vi "SeqnRead.vi"(8 "error in (no error)":errorcluster, 11 "File in":path) -> (0 "error out":errorcluster, 1 "Cohort List":cluster{string, i32}[](array[cluster]), 2 "Seqn out":refnum<class "Sequence.lvclass">)   [LabVIEW 2012, in "Sequence.lvclass"]
uses:
  Sequence.lvclass
  Cohort.lvclass
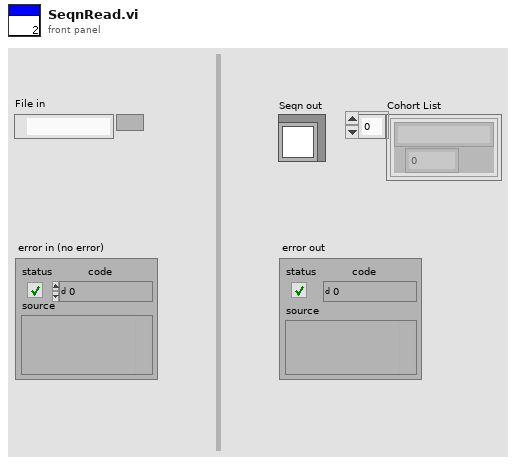
[diagram p1: front panel]
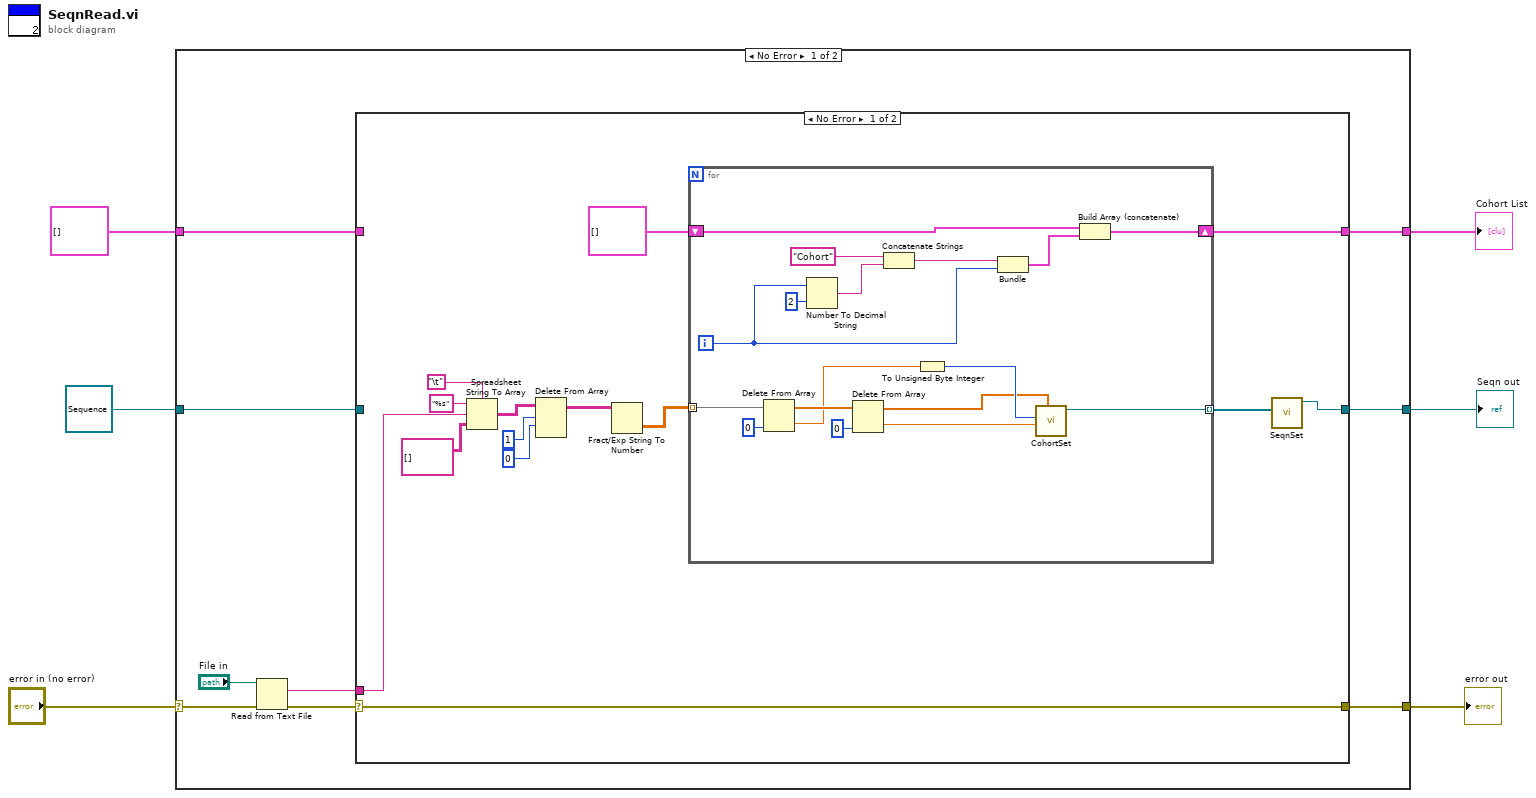
[diagram p0: block diagram]
diagram:
  n1 = case shown="No Error" "error in (no error)" {
    selector: "error in (no error)" -> [w11 w52]
    tunnel: [w12 w52] -> w5
    tunnel: [w10 w50] -> w4
    tunnel: [w9 w51] -> w3
    tunnel: cluster{string, i32}[] [] -> [w8 w51]
    tunnel: refnum<class "Sequence.lvclass"> refnum ("Sequence.lvclass") -> [w7 w50]
    frame No Error {
      n2 = Read from Text File(file (use dialog)="File in", error in=w11) -> (text=w15:string, error out=w14:errorcluster)  [unwired: 2 in, 2 out]
      n3 = case shown="No Error" w14 {
        selector: w14 -> [w26 w49]
        tunnel: [w29 w48] -> w9
        tunnel: w15 -> [w27 _]
        tunnel: [w17 w47] -> w10
        tunnel: [w26 w49] -> w12
        tunnel: w8 -> [_ w48]
        tunnel: w7 -> [_ w47]
        frame No Error {
          n4 = Spreadsheet String To Array(delimiter (Tab)="\t", format string="%s", spreadsheet string=w27, array type (2D Dbl)=string[][] []) -> (array=w23:string[][])
          n5 = Delete From Array(array=w23, length=1, index (row)=0) -> (array with subset deleted=w20:string[][])  [unwired: 1 in, 1 out]
          n6 = Fract/Exp String To Number(string=w20) -> (number=w19:dbl[][])  [unwired: 3 in, 1 out]
          n7 = for {
            shift-right: [w43] -> w29
            shift-left: cluster{string, i32}[] [] -> [w42]
            tunnel: w19 -> [w38] mode=indexing
            tunnel: [w33] -> w18 mode=indexing
            i -> [w39]
            n8 = Delete From Array(array=w38, index=0) -> (deleted portion=w34:dbl, array with subset deleted=w35:dbl[])  [unwired: 1 in]
            n9 = Number To Decimal String(number=w39, width (-)=i16 2) -> (decimal integer string=w44:string)
            n10 = Delete From Array(array=w35, index=0) -> (deleted portion=w31:dbl, array with subset deleted=w30:dbl[])  [unwired: 1 in]
            n11 = Concatenate Strings("Cohort", w44) -> (w41:string)
            n12 = To Unsigned Byte Integer(number=w34) -> (unsigned 8bit integer=w32:u8)
            n13 = Bundle(w41, w39) -> (w40:cluster{string, i32})  [unwired: 1 in]
            n14 = call "CohortSet.vi"("Set Electrodes"=w30, "Set Pulse Width"=w31, "Set Pulse Frequency"=w32) -> ("Cohort out"=w33:refnum<class "Cohort.lvclass">)  [unwired: 7 in, 1 out]
            n15 = Build Array (concatenate)(w42, w40) -> (w43:cluster{string, i32}[])
          }
          n16 = call "SeqnSet.vi"("Sequence"=w18) -> ("Sequence out"=w17:refnum<class "Sequence.lvclass">)  [unwired: 8 in, 1 out]
        }
        frame Error {
        }
      }
    }
    frame Error {
    }
  }
  "error out" <- w5
  "Seqn out" <- w4
  "Cohort List" <- w3
